vi "Step_state_conditionally.vi"(10 "Time passed":bool, 11 "State in":T1) -> (3 "State out":T1)   [LabVIEW 2016]
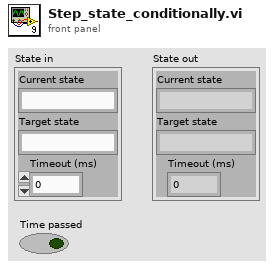
[diagram p1: front panel]
types:
  T1 = cluster{"Current state":string, "Target state":string, "Timeout (ms)":dbl}
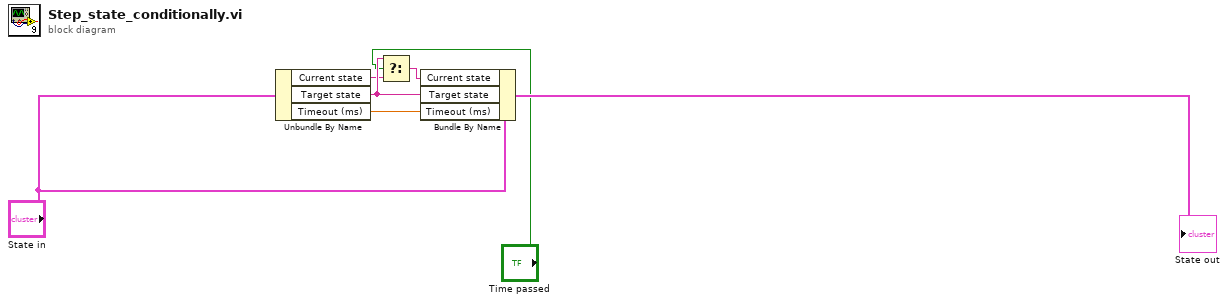
[diagram p0: block diagram]
diagram:
  n1 = Unbundle By Name("State in") -> ("Current state"=w2:string, "Target state"=w5:string, "Timeout (ms)"=w6:dbl)
  n2 = Select(t=w5, s="Time passed", f=w2) -> (s? t:f=w3:string)
  n3 = Bundle By Name(cluster="State in", "Current state"=w3, "Target state"=w5, "Timeout (ms)"=w6) -> (→"State out":T1)
